vi "calcOffset.vi"(0 "data in":dbl[](array[numeric]), 9 "offset":bool) -> (4 "data out":dbl[](array[numeric]), 8 "max":dbl, 10 "min":dbl, 15 "offset":dbl)   [LabVIEW 2023]
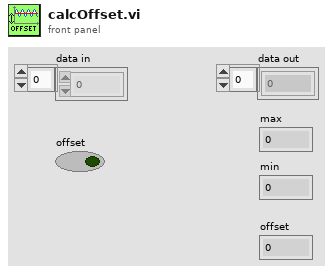
[diagram p1: front panel]
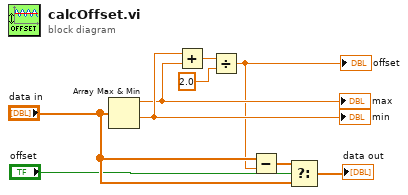
[diagram p0: block diagram]
diagram:
  n1 = Array Max & Min(array="data in") -> (max value=w7:dbl, min value=w8:dbl)  [unwired: 2 out]
  "min" <- w8
  "max" <- w7
  n2 = Add(x=w8, y=w7) -> (x+y=w9:dbl)
  n3 = Divide(x=w9, y=2.0 ("x")) -> (x/y=w3:dbl)
  "offset" <- w3
  n4 = Subtract(x="data in", y=w3) -> (x-y=w5:dbl[])
  n5 = Select(t=w5, s="offset", f="data in") -> (s? t:f=→"data out":dbl[])
